vi "Simple Reader.vi"(8 "error in (no error)":errorcluster, 11 "Fluke 1586A Driver in":refnum<class "Fluke 1586A Driver.lvclass">) -> (0 "error out":errorcluster, 2 "Signals":dbl[](array[numeric]), 3 "Fluke 1586A Driver out":refnum<class "Fluke 1586A Driver.lvclass">)   [LabVIEW 2021, in "Fluke 1586A Driver.lvclass"]
uses:
  Fluke 1586A Driver.lvclass
  C:/GitHub/NHMFL_Core/Libraries/Instruments/VISA Instrument/VISA Instrument.lvclass
  VISA Instrument/VISA Instrument.lvclass/VISA Instrument.ctl
  Fluke 1586A Driver.lvclass/Fluke 1586A Driver.ctl
  VISA Instrument/Read VISA resource.vi
  VISA Instrument/Write VISA resource.vi
  GPIB/VISA  Send Receive.vi
  Simple VISA Reader/Simple VISA Reader Driver.lvclass
panel:
  out "x-y":u32
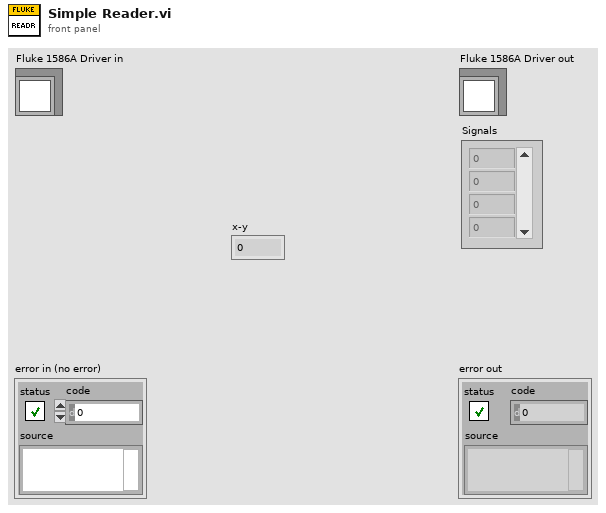
[diagram p1: front panel]
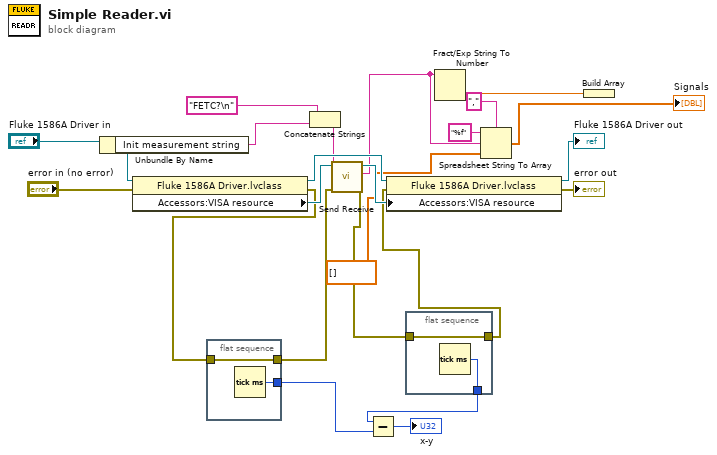
[diagram p0: block diagram]
diagram:
  n1 = Unbundle By Name("Fluke 1586A Driver in") -> ("Init measurement string"=w8:string)
  n2 = property class="Fluke 1586A Driver.lvclass"(reference="Fluke 1586A Driver in", error in="error in (no error)") -> (reference out=w20:refnum<class "Fluke 1586A Driver.lvclass">, error out=w7:errorcluster, "Accessors:VISA resource"=w22:refnum<visa-resource-name>)
  n3 = flat-sequence {
    tunnel: w7 -> [w25]
    tunnel: [w25] -> w6
    tunnel: [w24] -> w2
    frame #0 {
      n4 = Tick Count (ms)() -> (millisecond timer value=w24:u32)
    }
  }
  n5 = Concatenate Strings("FETC?\n" ("data string in"), w8) -> (w10:string)
  n6 = call-poly "Send Receive.vi"("error in (no error)"=w6, "data string in"=w10, "VISA Resource Name"=w22) -> ("error out"=w5:errorcluster, "data string out"=w15:string, "VISA Resource Name Out"=w19:refnum<visa-resource-name>)  [unwired: 6 in]
  n7 = Subtract(x=w3, y=w2) -> (x-y=→"x-y":u32)
  n8 = property class="Fluke 1586A Driver.lvclass"(reference=w20, error in=w4, "Accessors:VISA resource"=w19) -> (reference out=→"Fluke 1586A Driver out":refnum<class "Fluke 1586A Driver.lvclass">, error out=→"error out":errorcluster)
  n9 = flat-sequence {
    tunnel: w5 -> [w27]
    tunnel: [w27] -> w4
    tunnel: [w26] -> w3
    frame #0 {
      n10 = Tick Count (ms)() -> (millisecond timer value=w26:u32)
    }
  }
  n11 = Fract/Exp String To Number(string=w15) -> (number=w16:dbl)  [unwired: 3 in, 1 out]
  n12 = Spreadsheet String To Array(delimiter (Tab)=",", format string="%f", spreadsheet string=w15, array type (2D Dbl)=dbl[] []) -> (array=→"Signals":dbl[])
  n13 = Build Array(w16) -> ()  [unwired: 1 out]
